vi "Untitled 2.vi"() -> ()   [LabVIEW 2017]
uses:
  <vilib>/Platform/TimedLoop/XDataNode/timing_clust.ctl
  <vilib>/Platform/TimedLoop/XDataNode/nitl_modes.ctl
  <vilib>/Platform/TimedLoop/XDataNode/wakeup.ctl
  <vilib>/FPGAPlugInAG/cRIO-9065/niLvFpga_Open_cRIO-9065.vi
  <vilib>/rvi/interface/common/dynamic/niFpgaDynamicAddResources.vi
  <vilib>/Utility/error.llb/Error Cluster From Error Code.vi
  <vilib>/rvi/errors/niLvFpgaAdjustHostInterfaceError.vi
  <vilib>/FPGAPlugInAG/Dynamic/niLvFpga_Run_Dynamic.vi
  <vilib>/FPGAPlugInAG/Dynamic/niLvFpga_Abort_Dynamic.vi
  <vilib>/rvi/interface/nirviOpenFPGA/nirviOpenFPGA.xnode
  FPGA Bitfiles/fpgaproject_FPGATarget_fpgamain2_8UW6JkLDP9I.lvbitx
  fpga main2.vi
  <vilib>/rvi/interface/nirviMethod/nirviMethod.xnode
  <vilib>/rvi/interface/nirviReadWriteControl/nirviReadWriteControl.xnode
  <vilib>/platform/TimedLoop/XDataNode/XDataNode.xnode
  NiFpgaLv.dll
  <vilib>/rvi/interface/Simulation/niFpgaSimulationCallBeginRW.vi
  <vilib>/Platform/TimedLoop/XDataNode/XDNodeRunTimeDep.lvlib
  <vilib>/FPGAPlugInAG/Dynamic/niLvFpga_StartFifo_Dynamic.vi
  <vilib>/rvi/errors/niLvFpgaMergeErrorWithErrorCode.vi
panel:
  out "Enocder Position":dbl[](graph)
  in  "Period":i64
  in  "stop":bool
  out "error out 2":errorcluster
  out "Real period":u32
  out "速率":dbl
  in  "Position Reset":bool
  out "Encoder Position":dbl format="%#_8g"
  out "error out":errorcluster
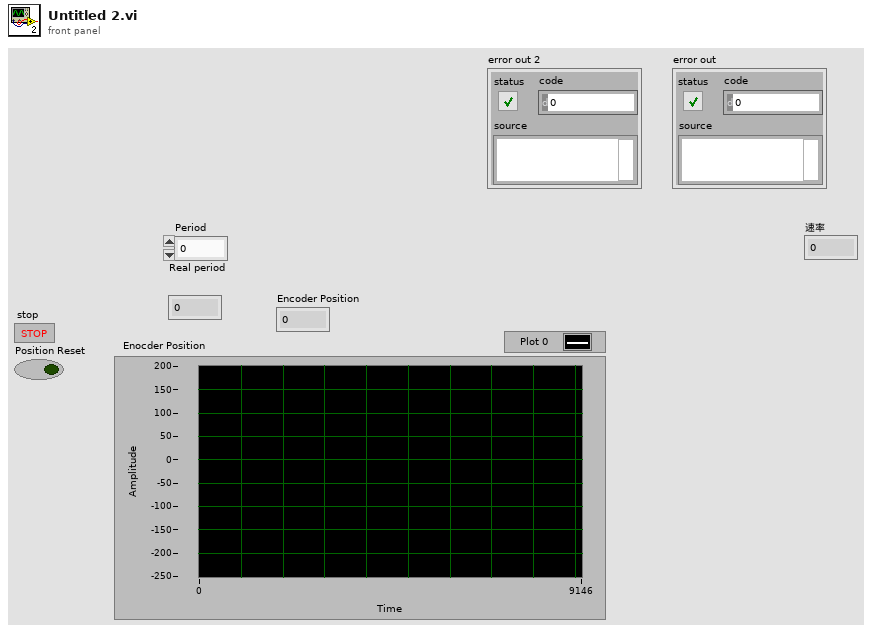
[diagram p1: front panel]
types:
  T1 = typedef "XDNodeRunTimeDep.lvlib/timing_clust.ctl" = cluster{"Expected End [f-1]":u64, "Actual End [f-1]":u64, "Finished Late? [f-1]":bool, "Expected End [i-1]":u64, "Actual End [i-1]":u64, "Finished Late? [i-1]":bool, "Expected Start [i]":u64, "Actual Start [i]":u64, "Expected Start [f]":u64, "Actual Start [f]":u64, "Source Name":string, "Structure Name":string, "Period":i64, "Deadline":i64, "Offset":i64, "Start":i64, "Priority":i32, "Timeout":i32, "Mode":T2, "Wakeup Reason":T3, "Error":errorcluster, "Source Type":string, "Secondary Source Type":string, "Global End Time":u64, "Global Start Time":u64, "Frame Duration":u64, "Iteration Duration":u64, "Assigned CPU":i32, "I/O Scan Engine Mode":u32}
  T2 = typedef "XDNodeRunTimeDep.lvlib/nitl_modes.ctl" = enum32{"No Change", "Process missed periods, maintain original phase", "Discard missed periods, maintain original phase", "Process missed periods, ignore original phase", "Discard missed periods, ignore original phase"}
  T3 = typedef "XDNodeRunTimeDep.lvlib/wakeup.ctl" = enum32{"Normal", "Aborted", "Asynchronous wakeup", "Timing source error", "Timed loop error", "Timeout"}
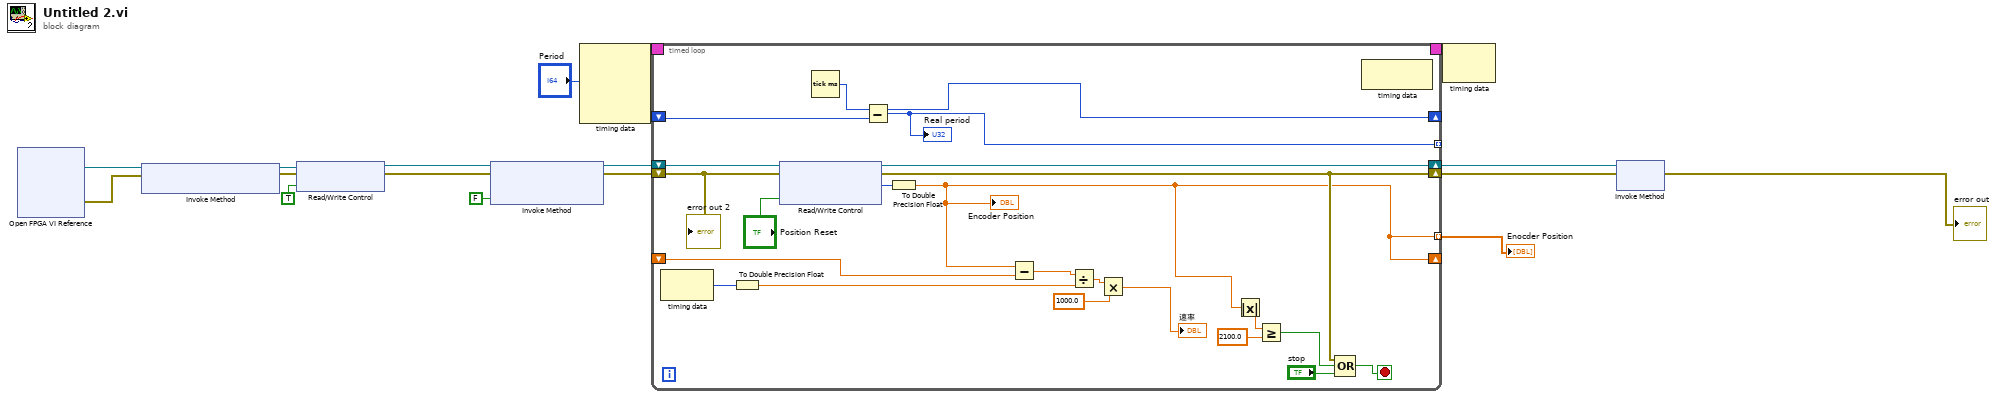
[diagram p0: block diagram]
diagram:
  n1 = xnode "Open FPGA VI Reference"() -> ("FPGA VI Reference Out"=w5:refnum<k20>, "error out"=w4:errorcluster)  [unwired: 2 in]
  n2 = xnode "Invoke Method"("FPGA VI Reference In"=w5, "error in"=w4) -> ("FPGA VI Reference Out"=w7:refnum<k20>, "error out"=w6:errorcluster)
  n3 = xnode "Read/Write Control"("FPGA VI Reference In"=w7, "error in"=w6, "Position Reset"=TRUE) -> ("FPGA VI Reference Out"=w11:refnum<k20>, "error out"=w10:errorcluster)
  n4 = xnode "Invoke Method"("FPGA VI Reference In"=w11, "error in"=w10, "Wait Until Done (F)"=FALSE) -> ("FPGA VI Reference Out"=w13:refnum<k20>, "error out"=w12:errorcluster)
  n5 = node-c288("Period") -> (w17:T1)  [unwired: 3 in]
  n6 = timed-loop {
    shift-right: [w34] -> w15
    shift-left: w13 -> [w32]
    shift-right: [w27] -> w14
    shift-left: w12 -> [w35]
    shift-right: [w38] -> _
    shift-left: _ -> [w39]
    timing: w17 -> [_]
    timing-out: [_] -> w16
    tunnel: [w37] -> _ mode=indexing
    shift-right: [w18] -> _
    shift-left: _ -> [w33]
    tunnel: [w18] -> w1 mode=indexing
    stop <- w29 stop-if-true
    n7 = node-c288() -> (w23:i64)  [unwired: 1 in]
    n8 = To Double Precision Float(number=w23) -> (double precision float=w22:dbl)
    n9 = xnode "Read/Write Control"("FPGA VI Reference In"=w32, "error in"=w35, "Position Reset"="Position Reset") -> ("FPGA VI Reference Out"=w34:refnum<k20>, "error out"=w27:errorcluster, "Position (Counts)"=w24:i32)
    n10 = Tick Count (ms)() -> (millisecond timer value=w38:u32)
    n11 = Subtract(x=w38, y=w39) -> (x-y=w37:u32)
    "Real period" <- w37
    n12 = To Double Precision Float(number=w24) -> (double precision float=w18:dbl)
    "Encoder Position" <- w18
    n13 = Subtract(x=w18, y=w33) -> (x-y=w36:dbl)
    n14 = Divide(x=w36, y=w22) -> (x/y=w21:dbl)
    n15 = Multiply(x=w21, y=1000.0) -> (x*y=→"速率":dbl)
    n16 = Absolute Value(x=w18) -> (abs(x)=w19:dbl)
    n17 = Greater Or Equal?(x=w19, y=2100.0) -> (x >= y?=w26:bool)
    n18 = Compound Arithmetic op=OR(w27, w26, "stop") -> (w29:bool)
    n19 = node-c288() -> ()  [unwired: 1 in, 1 out]
    "error out 2" <- w35
  }
  "Enocder Position" <- w1
  n20 = node-c288(w16) -> ()  [unwired: 1 out]
  n21 = xnode "Invoke Method"("FPGA VI Reference In"=w15, "error in"=w14) -> ("error out"=→"error out":errorcluster)  [unwired: 1 out]
